vi "Boiler Controller.vi"(8 "error in":errorcluster, 10 "Notifiers":T1, 11 "Message Queues":T2) -> (0 "error out":errorcluster)   [LabVIEW 2014]
uses:
  support/Message Queue/All Message Queues.ctl
  support/Message Queue/Message Cluster.ctl
  support/Notifiers/Notifiers.ctl
  <vilib>/Utility/error.llb/Error Cluster From Error Code.vi
  <vilib>/ErrorRing/Error Ring.xnode
  support/Message Queue/Message Queue.lvlib
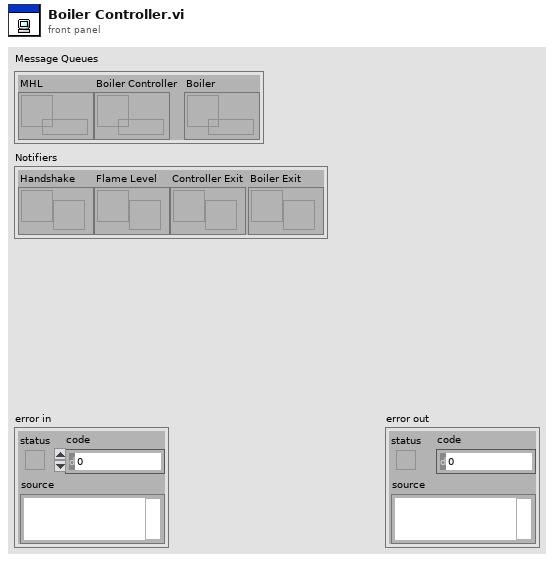
[diagram p1: front panel]
types:
  T1 = typedef "Notifiers.ctl" = cluster{"Handshake":refnum<notifier>, "Flame Level":refnum<notifier>, "Controller Exit":refnum<notifier>, "Boiler Exit":refnum<notifier>}
  T2 = typedef "Message Queue.lvlib/All Message Queues.ctl" = cluster{"MHL":refnum<queue>, "Boiler Controller":refnum<queue>, "Boiler":refnum<queue>}
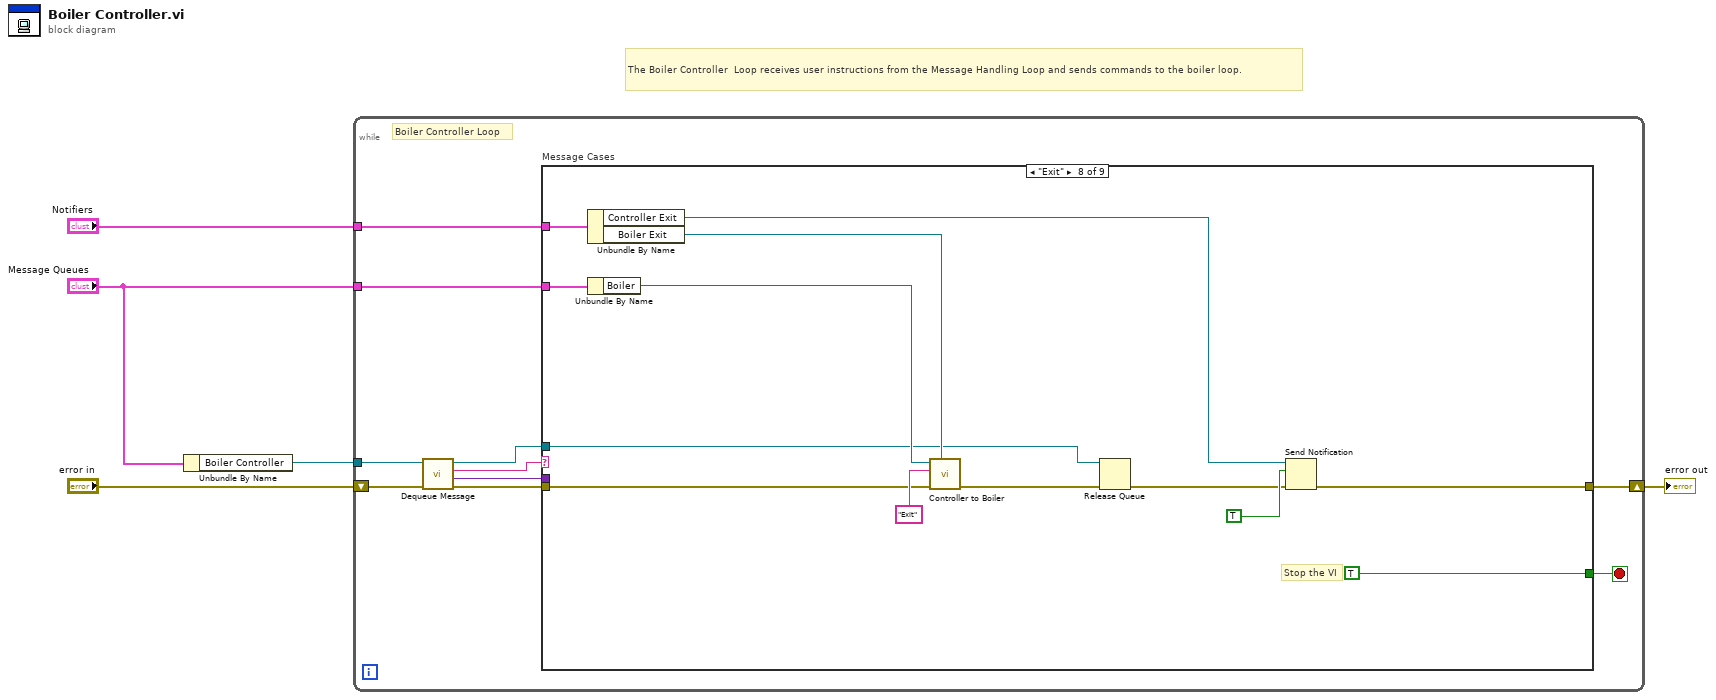
[diagram p0: block diagram]
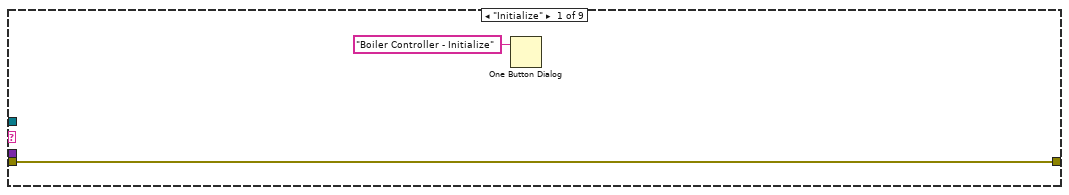
[diagram p2: hidden frame]
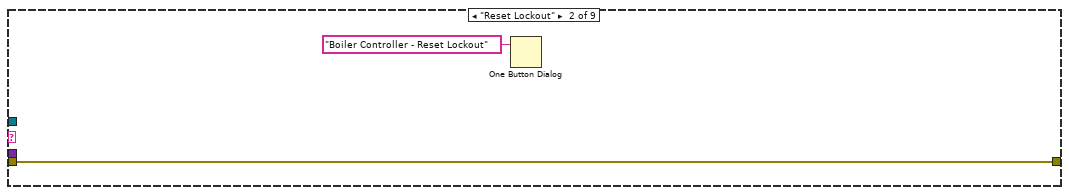
[diagram p3: hidden frame]
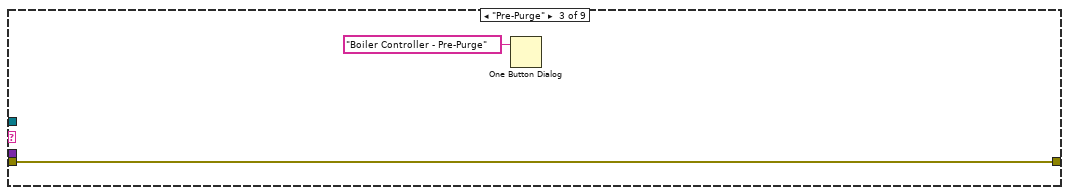
[diagram p4: hidden frame]
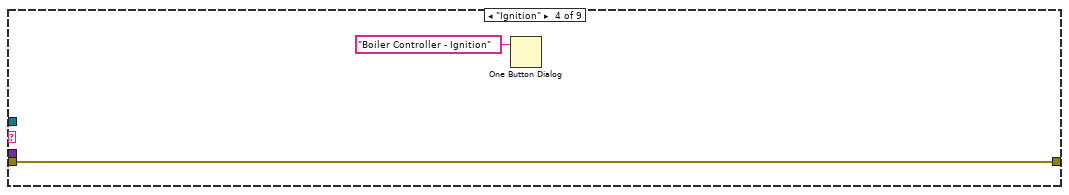
[diagram p5: hidden frame]
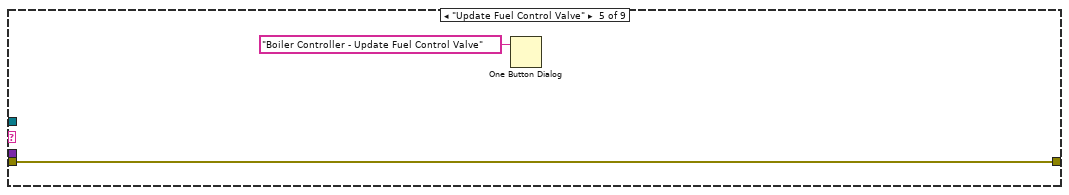
[diagram p6: hidden frame]
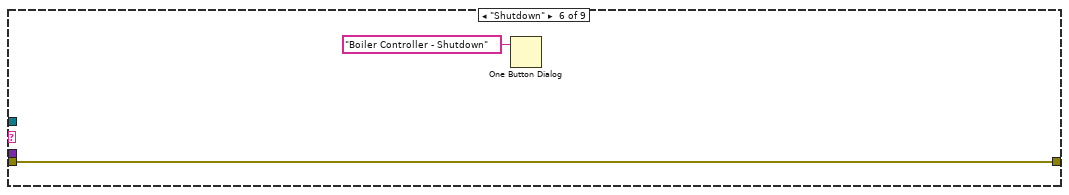
[diagram p7: hidden frame]
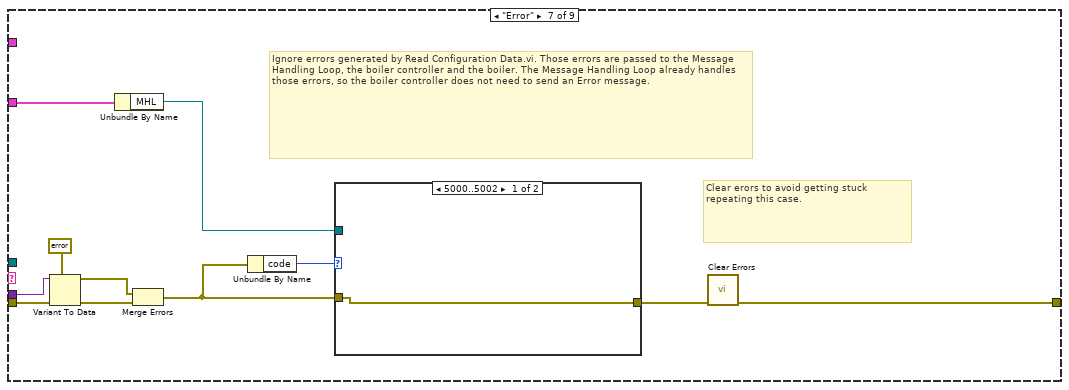
[diagram p8: hidden frame]
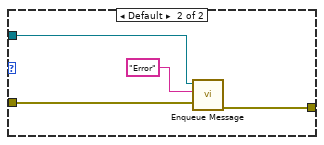
[diagram p9: hidden frame]
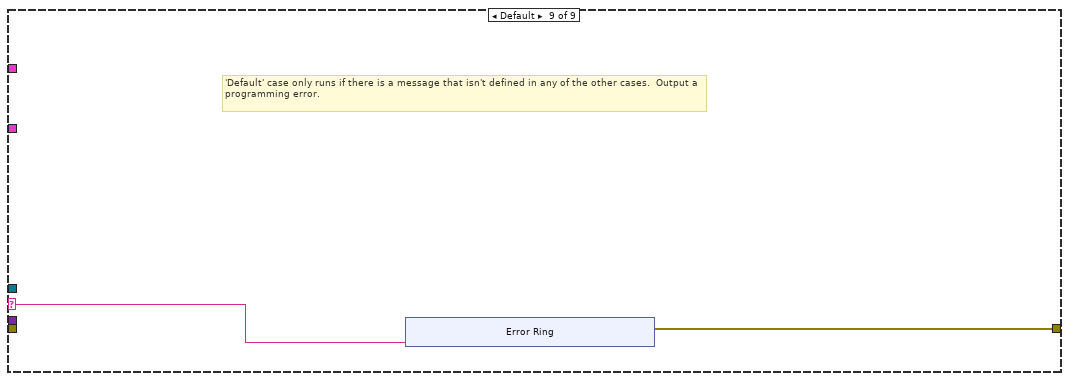
[diagram p10: hidden frame]
diagram:
  # "The Boiler Controller  Loop receives user instructions from the Message Handling Loop and sends commands to the boiler loop."
  n1 = Unbundle By Name("Message Queues") -> ("Boiler Controller"=w3:refnum<queue>)
  n2 = while {
    tunnel: w3 -> [w9]
    shift-right: [w8] -> w5
    shift-left: "error in" -> [w14]
    tunnel: "Message Queues" -> [w7]
    tunnel: "Notifiers" -> [w6]
    stop <- w15 stop-if-true
    # "Boiler Controller Loop"
    n3 = call "Dequeue Message.vi"("error in (no error)"=w14, "Message Queue"=w9) -> ("error out"=w13:errorcluster, "Message Data"=w11:variant, "Message"=w12:string, "dup Message Queue"=w10:refnum<queue>)  [unwired: 6 in]
    n4 = case "Message Cases" shown="\"Exit\"" w12 {
      selector: w12 -> [_ _ _ _ _ _ _ _ w57]
      tunnel: w10 -> [_ _ _ _ _ _ _ w49 _]
      tunnel: w13 -> [w17 w19 w21 w23 w25 w27 w36 w48 _]
      tunnel: [w17 w19 w21 w23 w25 w27 w30 w46 w58] -> w8
      tunnel: [_ _ _ _ _ _ _ TRUE _] -> w15
      tunnel: w11 -> [_ _ _ _ _ _ w34 _ _]
      tunnel: w7 -> [_ _ _ _ _ _ w38 w45 _]
      tunnel: w6 -> [_ _ _ _ _ _ _ w44 _]
      frame "Initialize" {
        n5 = One Button Dialog(message="Boiler Controller - Initialize") -> ()  [unwired: 1 in, 1 out]
      }
      frame "Reset Lockout" {
        n6 = One Button Dialog(message="Boiler Controller - Reset Lockout") -> ()  [unwired: 1 in, 1 out]
      }
      frame "Pre-Purge" {
        n7 = One Button Dialog(message="Boiler Controller - Pre-Purge") -> ()  [unwired: 1 in, 1 out]
      }
      frame "Ignition" {
        n8 = One Button Dialog(message="Boiler Controller - Ignition") -> ()  [unwired: 1 in, 1 out]
      }
      frame "Update Fuel Control Valve" {
        n9 = One Button Dialog(message="Boiler Controller - Update Fuel Control Valve") -> ()  [unwired: 1 in, 1 out]
      }
      frame "Shutdown" {
        n10 = One Button Dialog(message="Boiler Controller - Shutdown") -> ()  [unwired: 1 in, 1 out]
      }
      frame "Error" {
        # "Ignore errors generated by Read Configuration Data.vi. Those errors are passed to the Message Handling Loop, the boiler controller and the boiler. The Message Handling Loop already handles those errors, so the boiler controller does not need to send an Error message."
        # "Clear erors to avoid getting stuck repeating this case."
        n11 = Variant To Data(error in=w36, type=errorcluster {"status"=FALSE, "code"=0, "source"=""} ("error out"), Variant=w34) -> (data=w32:errorcluster, error out=w33:errorcluster)
        n12 = Unbundle By Name(w38) -> ("MHL"=w37:refnum<queue>)
        n13 = Merge Errors(w32, w33) -> (w29:errorcluster)
        n14 = Unbundle By Name(w29) -> ("code"=w28:i32)
        n15 = case shown="5000..5002" w28 {
          tunnel: w37 -> [_ w42]
          tunnel: [w39 w41] -> w31
          tunnel: w29 -> [w39 w40]
          frame 5000..5002 {
          }
          frame Default {
            n16 = call "Enqueue Message.vi"("Message Data"=w40, "Message"="Error", "Message Queue"=w42) -> ("error out"=w41:errorcluster)  [unwired: 7 in, 1 out]
          }
        }
        n17 = call <vilib>:"Clear Errors.vi"("error in (no error)"=w31) -> ("error out"=w30:errorcluster)  [unwired: 5 in, 1 out]
      }
      frame "Exit" {
        # "Stop the VI"
        n18 = Unbundle By Name(w44) -> ("Controller Exit"=w51:refnum<notifier>, "Boiler Exit"=w53:refnum<notifier>)
        n19 = Unbundle By Name(w45) -> ("Boiler"=w50:refnum<queue>)
        n20 = call "Controller to Boiler.vi"("Notifier"=w53, "error in"=w48, "Message"="Exit", "Boiler Queue in"=w50) -> ("error out"=w56:errorcluster)  [unwired: 5 in, 2 out]
        n21 = Release Queue(queue=w49, error in (no error)=w56) -> (error out=w52:errorcluster)  [unwired: 1 in, 2 out]
        n22 = Send Notification(notification=TRUE, notifier=w51, error in (no error)=w52) -> (error out=w46:errorcluster)  [unwired: 1 out]
      }
      frame Default {
        # "'Default' case only runs if there is a message that isn't defined in any of the other cases.  Output a programming error."
        n23 = xnode "Error Ring"("parameter 0"=w57) -> ("error out"=w58:errorcluster)
      }
    }
  }
  "error out" <- w5
